vi "GT Pt Ao.vi"(5 "fifo":i16, 6 "value":dbl, 7 "index":i16, 8 "error in (no error)":errorcluster caption="错误输入（无错误）", 9 "aoType":i16, 10 "profile":i16, 11 "cardNum":i16) -> (0 "error out":errorcluster caption="错误输出", 3 "function return":i16)   [LabVIEW 2014, in "gts.lvlib"]
doc: "GT_API GT_PtAo(short cardNum,short profile,short aoType,short index,double value,short fifo);"
uses:
  gts.lvlib
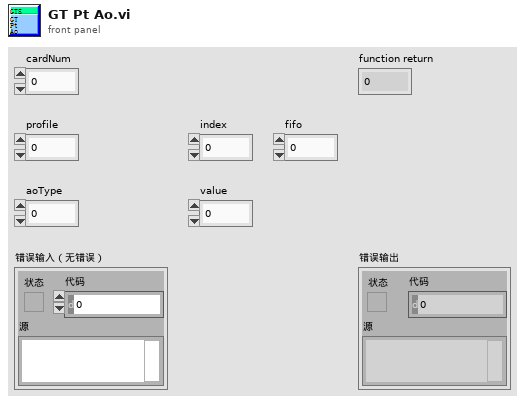
[diagram p1: front panel]
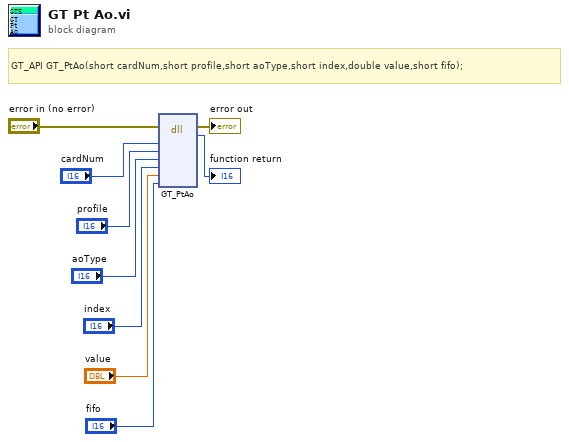
[diagram p0: block diagram]
diagram:
  # "GT_API GT_PtAo(short cardNum,short profile,short aoType,short index,double value,short fifo);"
  n1 = dll-call lib="PTH2habs D固高科技资料GTS控制卡GTS卡18年上半年资料dllVC32bit\nmulti_cardgts.*" fn="GT_PtAo"(error in="error in (no error)", "cardNum"="cardNum", "profile"="profile", "aoType"="aoType", "index"="index", "value"="value", "fifo"="fifo") -> (error out=→"error out":errorcluster, →"function return":i16)  [unwired: 8 in, 1 out]
